vi "BRig_dataAnalog_init.vi"() -> (3 "output_dataAnalog":u16[][](array[numeric]))   [LabVIEW 2014]
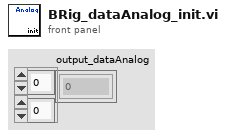
[diagram p1: front panel]
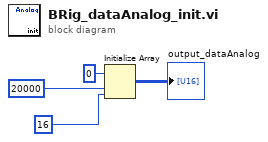
[diagram p0: block diagram]
diagram:
  n1 = Initialize Array(u16 0 ("element"), 20000 ("dimension size"), 16 ("dimension size")) -> (→"output_dataAnalog":u16[][])
